vi "Controller Open Ethercat Variables.vi"(8 "error in (no error)":errorcluster, 11 "FOFB Configuration":T3={"FOFB Parameters"={"Network"={"FOFB Controller IP"="", "LNLS Control Network IP"="", "LNLS Control Network Power Supplies TCP Port"=0, "LNLS Control Network FOFB Configuration TCP Port"=0, "LNLS Control Network BPMs TCP Port"=0, "Monitoring Data TCP Port"=0, "Fast Archiver TCP Port"=0, "Fast Command TCP Port"=0, "TCP Listening Timeout"=0}, "Fast Acquisition"={"Sampling Period"=0, "Data Buffer Size"=0, "Monitoring Period"=0}, "Acquisition Network"=[], "Actuation Network"=[]}, "Number of Acquisition Chassis"=0, "Number of Actuation Chassis"=0, "Number of BPM Readings"=0, "BPM Reading Names"=[], "Selected BPM Readings"=[0, 1, 2, 3, 4, 5, 6, 7, 8, 9, 10, 11, 12, 13, 14, 15, 16, 17, 18, 19, 20, 21, 22, 23, 24, 25, 26, 27, 28, 29, 30, 31, 32, 33, 34, 35, 36, 37, 38, 39, 40, 41, 42, 43, 44, 45, 46, 47, 48, 49], "Number of Correctors"=0, "Corrector Names"=[], "Selected Correctors"=[0, 1, 2, 3, 4, 5, 6, 7, 8, 9, 10, 11, 12, 13, 14, 15, 16, 17, 18, 19, 20, 21, 22, 23, 24, 25, 26, 27, 28, 29, 30, 31, 32, 33, 34, 35, 36, 37, 38, 39, 40, 41, 42, 43, 44, 45, 46, 47, 48, 49], "Response Matrix"=[], "Reference Orbit"=[], "Correction Matrix"=[], "FPGA Filter Sets"=[], "Acquisition Chassis Names"=[], "Actuation Chassis Names"=[], "Acquisition Variables"=[], "Actuation Variables"=[], "PS Matrix Mapping"=[], "Inverse PS Matrix Mapping"=[], "BPM Matrix Mapping"=[], "Inverse BPM Matrix Mapping"=[], "BPM Planes"=[], "Corrector Planes"=[]}) -> (0 "error out":errorcluster, 2 "PS Variables":T1, 3 "BPM Variables":T2)   [LabVIEW 2011, in "Controller VIs.lvlib"]
doc: "Open references for all Acquisition and Actuation variables which are used to exchange data between the FOFB Controller and the Acquisition/Actuation chassis via the EtherCAT networks."
uses:
  Controller VIs.lvlib
  Types Definitions/Type FOFB Configuration.ctl
  Types Definitions/Type FOFB Parameters.ctl
  Types Definitions/Type Network Configuration.ctl
  Types Definitions/Type FA Configuration.ctl
  Types Definitions/Type Acquisition Network Configuration.ctl
  Types Definitions/Type Actuation Network Configuration.ctl
  Types Definitions/Type BPM Variables.ctl
  Types Definitions/Type PS Variables.ctl
  Type Definitions.lvlib
  XML VIs.lvlib
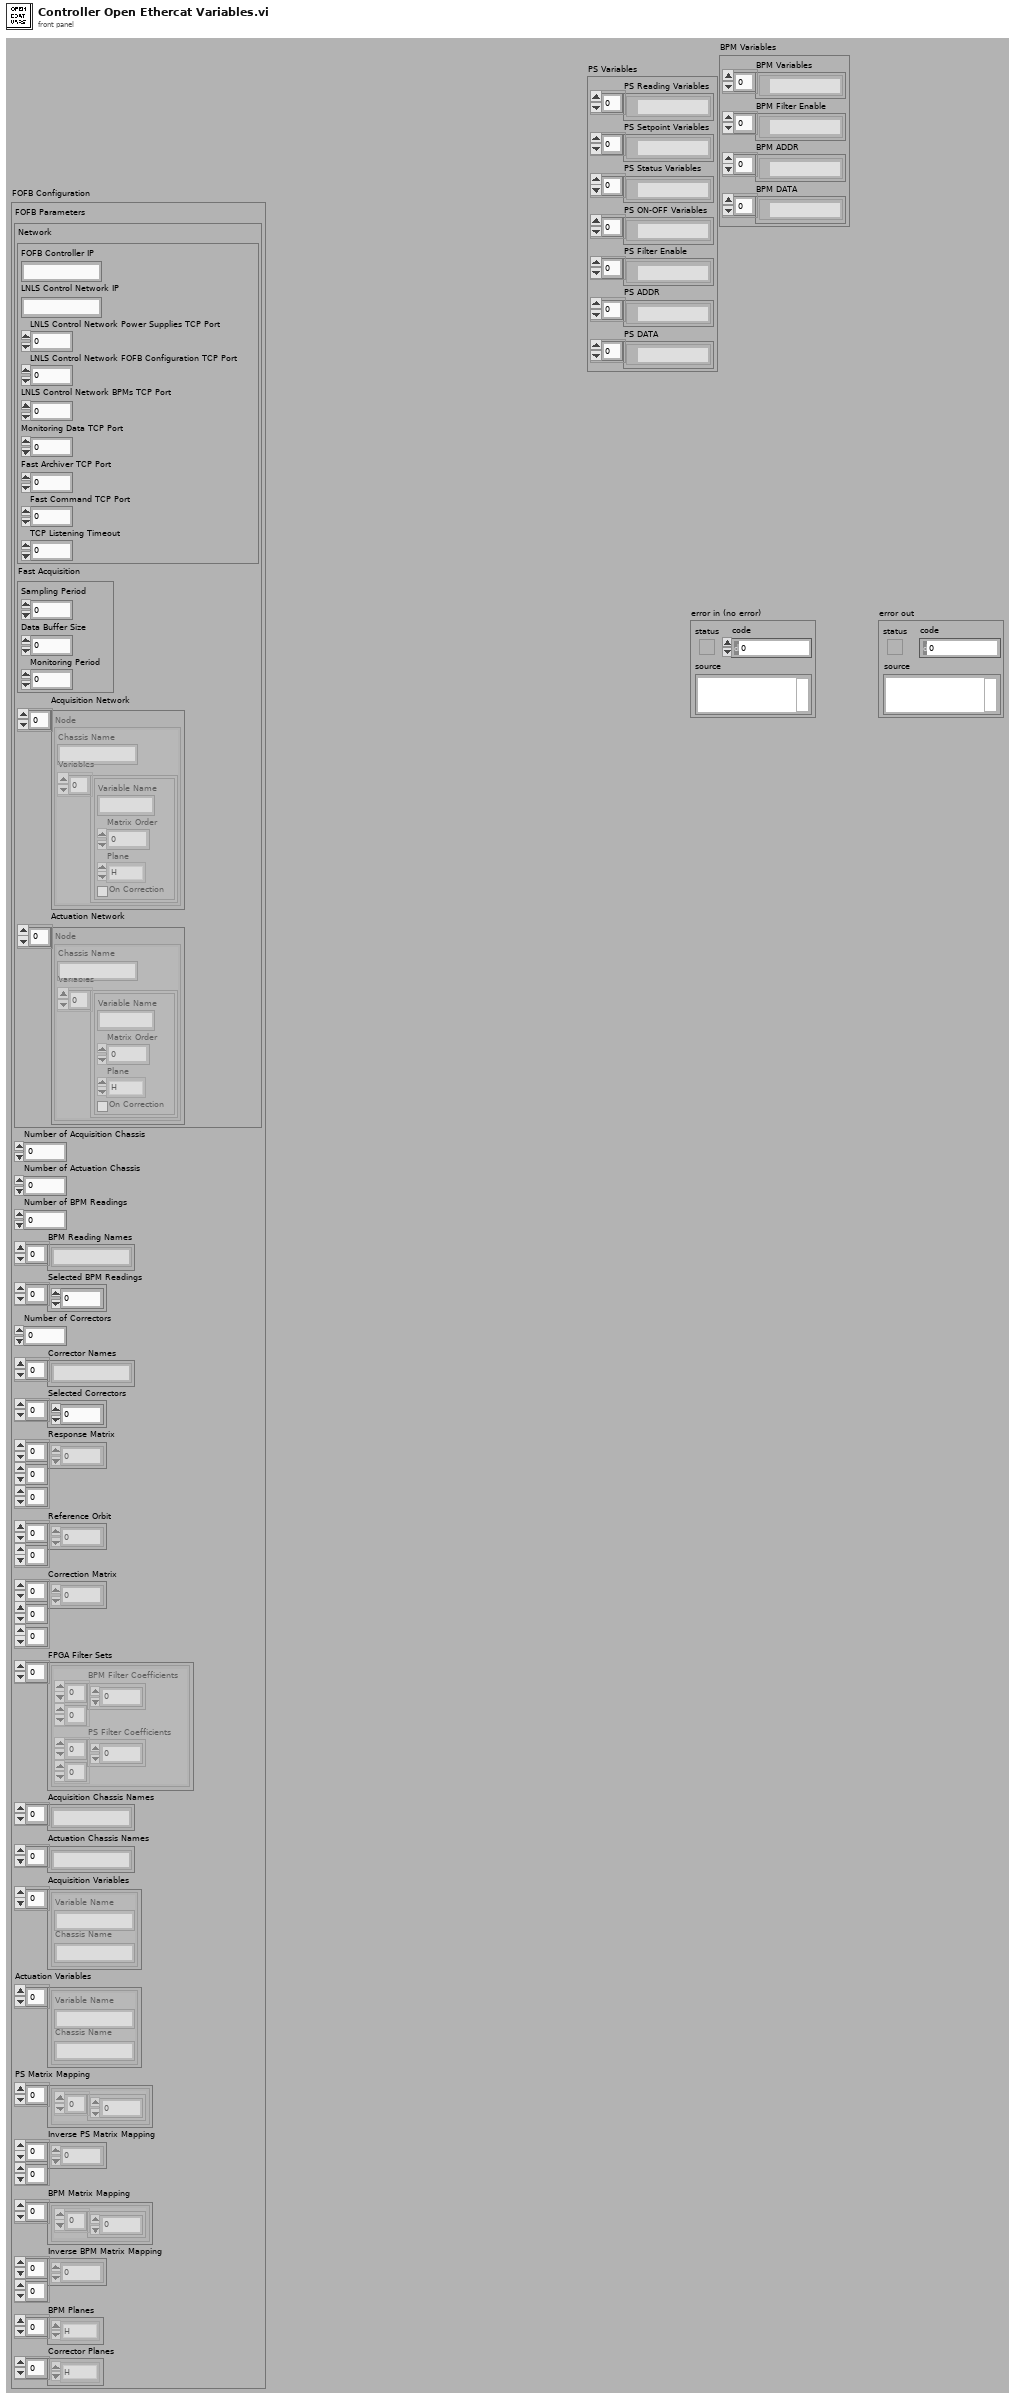
[diagram p1: front panel]
types:
  T1 = typedef "Type Definitions.lvlib/Type PS Variables.ctl" = cluster{"PS Reading Variables":refnum<k21>[], "PS Setpoint Variables":refnum<k21>[], "PS Status Variables":refnum<k21>[], "PS ON-OFF Variables":refnum<k21>[], "PS Filter Enable":refnum<k21>[], "PS ADDR":refnum<k21>[], "PS DATA":refnum<k21>[]}
  T2 = typedef "Type Definitions.lvlib/Type BPM Variables.ctl" = cluster{"BPM Variables":refnum<k21>[], "BPM Filter Enable":refnum<k21>[], "BPM ADDR":refnum<k21>[], "BPM DATA":refnum<k21>[]}
  T3 = typedef "Type Definitions.lvlib/Type FOFB Configuration.ctl" = cluster{"FOFB Parameters":T4, "Number of Acquisition Chassis":i32, "Number of Actuation Chassis":i32, "Number of BPM Readings":i32, "BPM Reading Names":string[], "Selected BPM Readings":u32[], "Number of Correctors":i32, "Corrector Names":string[], "Selected Correctors":u32[], "Response Matrix":dbl[][][], "Reference Orbit":dbl[][], "Correction Matrix":dbl[][][], "FPGA Filter Sets":cluster{"BPM Filter Coefficients":dbl[][], "PS Filter Coefficients":dbl[][]}[], "Acquisition Chassis Names":string[], "Actuation Chassis Names":string[], "Acquisition Variables":cluster{"Variable Name":string, "Chassis Name":string}[], "Actuation Variables":cluster{"Variable Name":string, "Chassis Name":string}[], "PS Matrix Mapping":cluster{u32[]}[], "Inverse PS Matrix Mapping":u32[][], "BPM Matrix Mapping":cluster{u32[]}[], "Inverse BPM Matrix Mapping":u32[][], "BPM Planes":enum8{"H", "V"}[], "Corrector Planes":enum8{"H", "V"}[]}
  T4 = typedef "Type Definitions.lvlib/Type FOFB Parameters.ctl" = cluster{"Network":T5, "Fast Acquisition":T6, "Acquisition Network":T7, "Actuation Network":T8}
  T5 = typedef "Type Definitions.lvlib/Type Network Configuration.ctl" = cluster{"FOFB Controller IP":string, "LNLS Control Network IP":string, "LNLS Control Network Power Supplies TCP Port":u16, "LNLS Control Network FOFB Configuration TCP Port":u16, "LNLS Control Network BPMs TCP Port":u16, "Monitoring Data TCP Port":u16, "Fast Archiver TCP Port":u16, "Fast Command TCP Port":u16, "TCP Listening Timeout":i32}
  T6 = typedef "Type Definitions.lvlib/Type FA Configuration.ctl" = cluster{"Sampling Period":u32, "Data Buffer Size":u32, "Monitoring Period":u32}
  T7 = typedef "Type Definitions.lvlib/Type Acquisition Network Configuration.ctl" = cluster{"Chassis Name":string, "Variables":cluster{"Variable Name":string, "Matrix Order":u32, "Plane":enum8{"H", "V"}, "On Correction":bool}[]}[]
  T8 = typedef "Type Definitions.lvlib/Type Actuation Network Configuration.ctl" = cluster{"Chassis Name":string, "Variables":cluster{"Variable Name":string, "Matrix Order":u32, "Plane":enum8{"H", "V"}, "On Correction":bool}[]}[]
  T9 = cluster{"Variable Name":string, "Chassis Name":string}[]
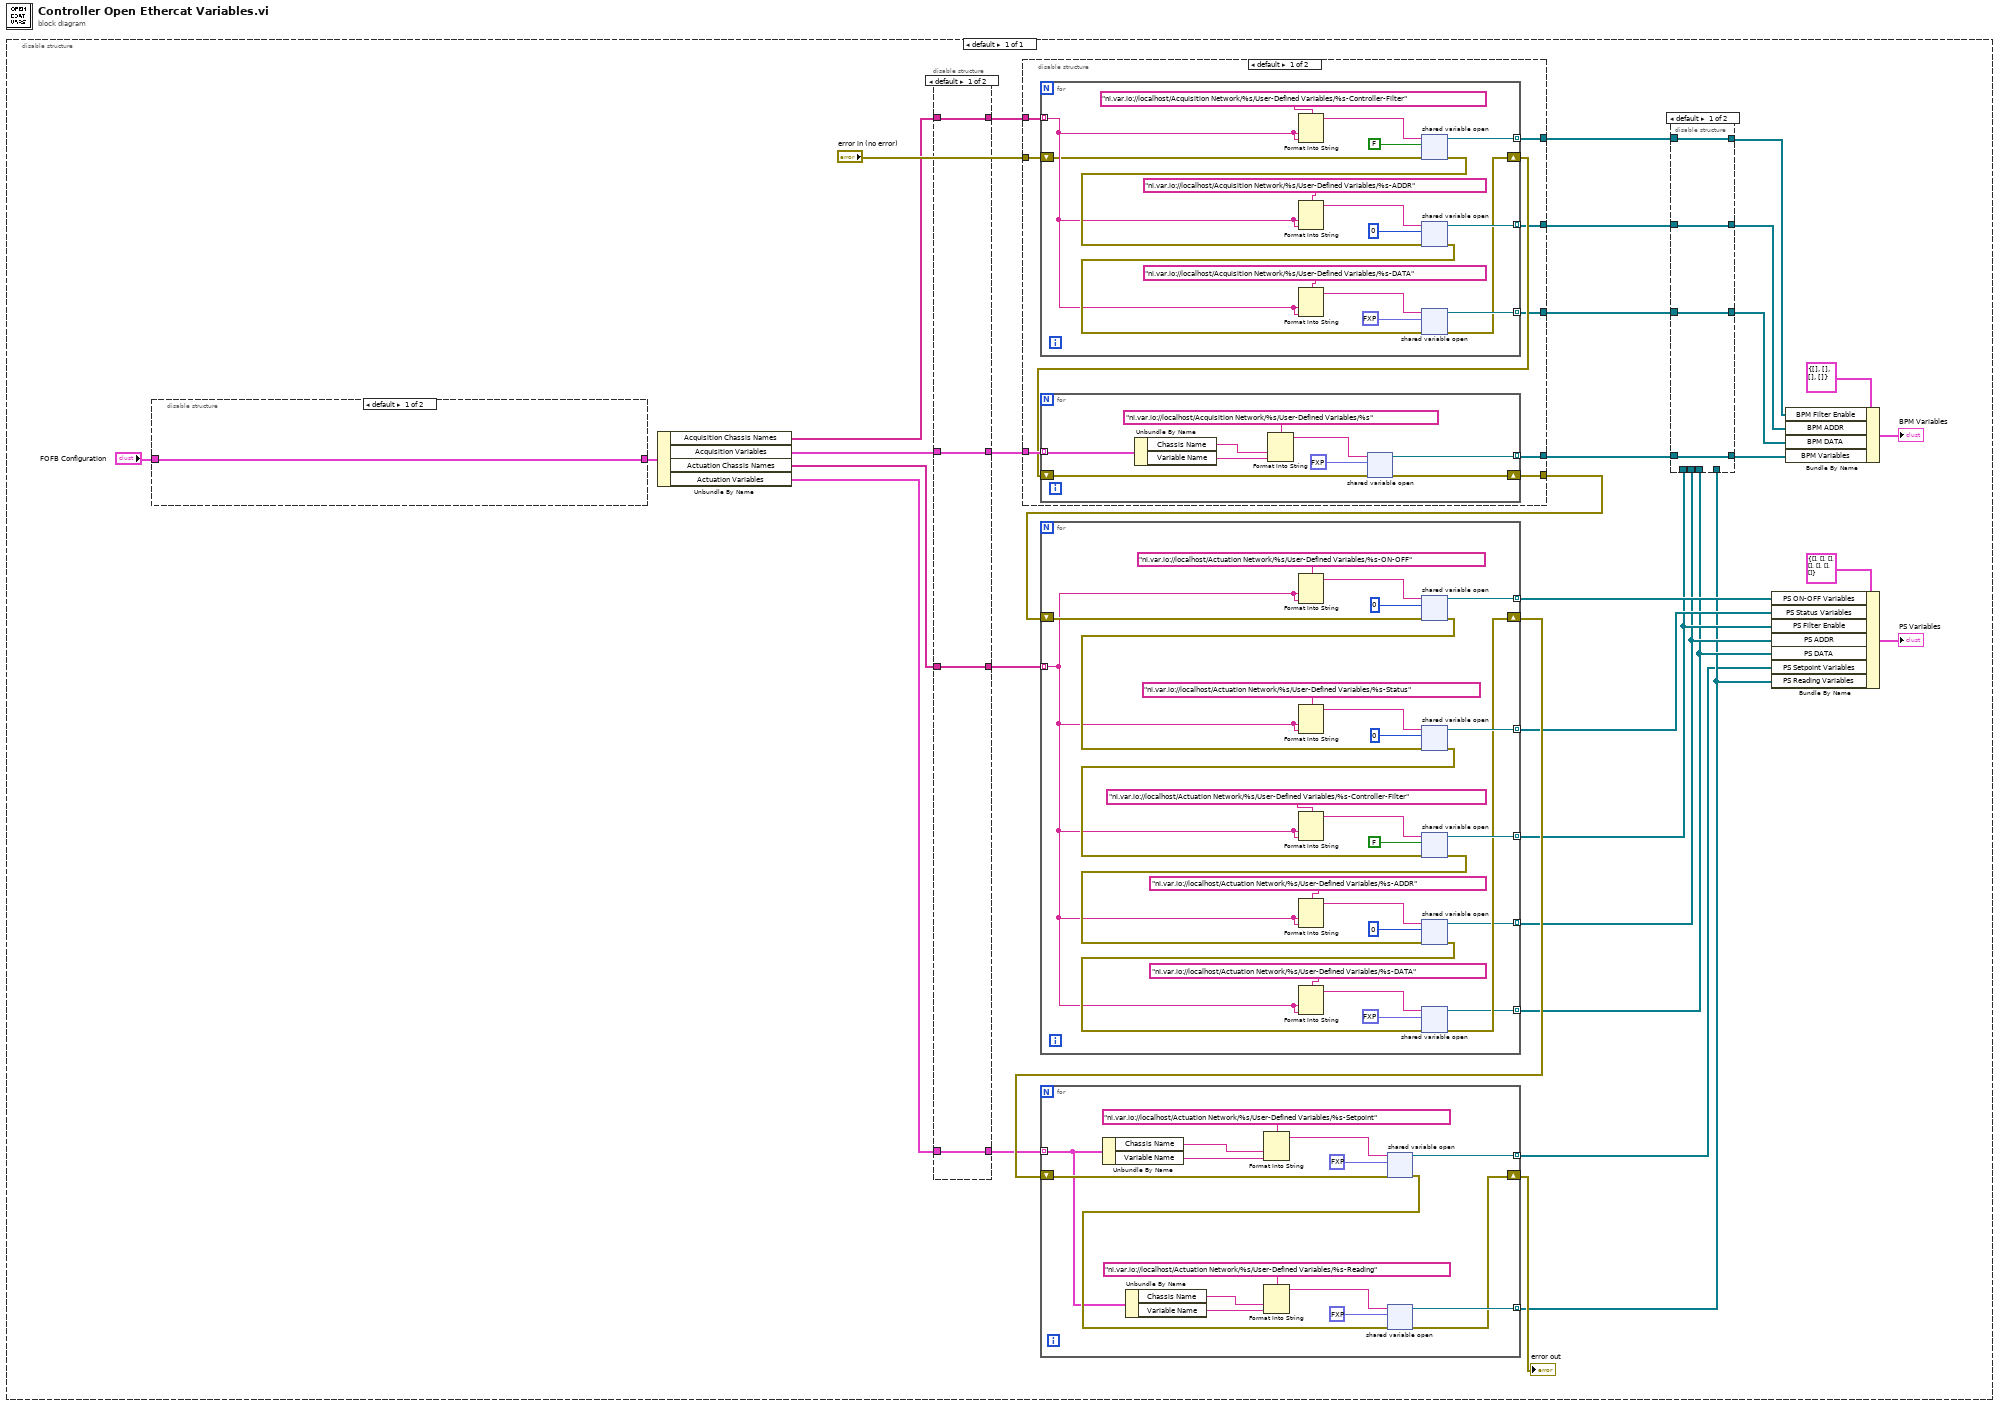
[diagram p0: block diagram]
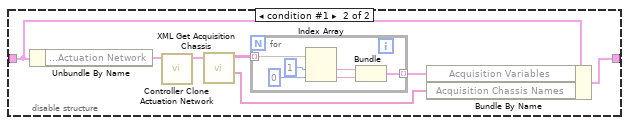
[diagram p2: hidden frame]
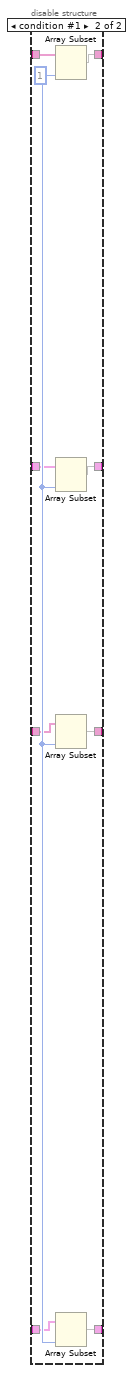
[diagram p3: hidden frame]
diagram:
  n1 = disable-structure shown="default" {
    frame Enabled {
      n2 = disable-structure shown="default" {
        disable-tunnel: "FOFB Configuration" -> [w34 w39]
        disable-tunnel: [w34 w36] -> w1
        frame condition #0 (active) {
        }
        frame condition #1 {
          n3 = Unbundle By Name(w39) -> ("FOFB Parameters.Actuation Network"=w41:T8)
          n4 = call "Controller Clone Actuation Network.vi"("Actuation Network"=w41) -> ("Acquisition Network"=w40:T7)  [unwired: 10 in]
          n5 = call "XML Get Acquisition Chassis.vi"("Acquisition Network"=w40) -> ("Acquisition Chassis Names"=w35:string[], "Acquisition Variable Names"=w38:string[][])  [unwired: 4 in, 5 out]
          n6 = for {
            tunnel: w38 -> [w46] mode=indexing
            tunnel: [w45] -> w37 mode=indexing
            n7 = Index Array(array=w46, index #1=1 ("index"), index #2=0 ("index")) -> (element #1=w42:string, element #2=w44:string)
            n8 = Bundle(w42, w44) -> (w45:cluster{string, string})  [unwired: 1 in]
          }
          n9 = Bundle By Name(cluster=w39, "Acquisition Variables"=w37, "Acquisition Chassis Names"=w35) -> (w36:T3)
        }
      }
      n10 = Unbundle By Name(w1) -> ("Acquisition Chassis Names"=w10:string[], "Acquisition Variables"=w8:T9, "Actuation Chassis Names"=w6:string[], "Actuation Variables"=w4:T9)
      n11 = disable-structure shown="default" {
        disable-tunnel: [w51 w59] -> w9
        disable-tunnel: w10 -> [w51 w60]
        disable-tunnel: [w50 w58] -> w7
        disable-tunnel: w8 -> [w50 w54]
        disable-tunnel: [w48 w57] -> w5
        disable-tunnel: [w49 w56] -> w3
        disable-tunnel: w4 -> [w49 w53]
        disable-tunnel: w6 -> [w48 w52]
        frame condition #0 (active) {
        }
        frame condition #1 {
          w55 = 1 ("length")
          n12 = Array Subset(array=w60, length=w55) -> (w59:string[])  [unwired: 1 in]
          n13 = Array Subset(array=w54, length=w55) -> (w58:T9)  [unwired: 1 in]
          n14 = Array Subset(array=w52, length=w55) -> (w57:string[])  [unwired: 1 in]
          n15 = Array Subset(array=w53, length=w55) -> (w56:T9)  [unwired: 1 in]
        }
      }
      n16 = disable-structure shown="default" {
        disable-tunnel: [w77 w104] -> w30
        disable-tunnel: w7 -> [w76 _]
        disable-tunnel: [w75 _] -> w25
        disable-tunnel: w9 -> [w74 _]
        disable-tunnel: "error in (no error)" -> [w73 w104]
        disable-tunnel: [w71 _] -> w20
        disable-tunnel: [w70 _] -> w19
        disable-tunnel: [w69 _] -> w18
        frame condition #0 (active) {
          n17 = for {
            shift-right: [w78] -> w72
            shift-left: w73 -> [w79]
            tunnel: w74 -> [w84] mode=indexing
            tunnel: [w94] -> w71 mode=indexing
            tunnel: [w81] -> w70 mode=indexing
            tunnel: [w80] -> w69 mode=indexing
            n18 = Format Into String(format string="ni.var.io://localhost/Acquisition Network/%s/User-Defined Variables/%s-Controller-Filter", w84, w84) -> (resulting string=w92:string)  [unwired: 2 in, 1 out]
            n19 = Format Into String(format string="ni.var.io://localhost/Acquisition Network/%s/User-Defined Variables/%s-ADDR", w84, w84) -> (resulting string=w90:string)  [unwired: 2 in, 1 out]
            n20 = Format Into String(format string="ni.var.io://localhost/Acquisition Network/%s/User-Defined Variables/%s-DATA", w84, w84) -> (resulting string=w87:string)  [unwired: 2 in, 1 out]
            n21 = shared-variable-open(w92, w79, FALSE) -> (w94:refnum<k21>, w85:errorcluster)  [unwired: 1 in]
            n22 = shared-variable-open(w90, w85, u16 0) -> (w81:refnum<k21>, w86:errorcluster)  [unwired: 1 in]
            n23 = shared-variable-open(w87, w86, fxp<+/-,22,4> 0.0) -> (w80:refnum<k21>, w78:errorcluster)  [unwired: 1 in]
          }
          n24 = for {
            tunnel: w76 -> [w97] mode=indexing
            shift-right: [w102] -> w77
            shift-left: w72 -> [w101]
            tunnel: [w100] -> w75 mode=indexing
            n25 = Unbundle By Name(w97) -> ("Chassis Name"=w96:string, "Variable Name"=w95:string)
            n26 = Format Into String(format string="ni.var.io://localhost/Acquisition Network/%s/User-Defined Variables/%s", w96, w95) -> (resulting string=w99:string)  [unwired: 2 in, 1 out]
            n27 = shared-variable-open(w99, w101, fxp<+/-,20,5> 0.0 ("BPM Data")) -> (w100:refnum<k21>, w102:errorcluster)  [unwired: 1 in]
          }
        }
        frame condition #1 {
        }
      }
      n28 = for {
        shift-right: [w112] -> w29
        shift-left: w30 -> [w124]
        tunnel: w5 -> [w109] mode=indexing
        tunnel: [w123] -> w17 mode=indexing
        tunnel: [w122] -> w16 mode=indexing
        tunnel: [w120] -> w15 mode=indexing
        tunnel: [w106] -> w14 mode=indexing
        tunnel: [w105] -> w13 mode=indexing
        n29 = Format Into String(format string="ni.var.io://localhost/Actuation Network/%s/User-Defined Variables/%s-ON-OFF", w109, w109) -> (resulting string=w131:string)  [unwired: 2 in, 1 out]
        n30 = Format Into String(format string="ni.var.io://localhost/Actuation Network/%s/User-Defined Variables/%s-Status", w109, w109) -> (resulting string=w128:string)  [unwired: 2 in, 1 out]
        n31 = Format Into String(format string="ni.var.io://localhost/Actuation Network/%s/User-Defined Variables/%s-Controller-Filter", w109, w109) -> (resulting string=w118:string)  [unwired: 2 in, 1 out]
        n32 = Format Into String(format string="ni.var.io://localhost/Actuation Network/%s/User-Defined Variables/%s-ADDR", w109, w109) -> (resulting string=w116:string)  [unwired: 2 in, 1 out]
        n33 = Format Into String(format string="ni.var.io://localhost/Actuation Network/%s/User-Defined Variables/%s-DATA", w109, w109) -> (resulting string=w113:string)  [unwired: 2 in, 1 out]
        n34 = shared-variable-open(w131, w124, u8 0) -> (w123:refnum<k21>, w127:errorcluster)  [unwired: 1 in]
        n35 = shared-variable-open(w128, w127, u8 0) -> (w122:refnum<k21>, w121:errorcluster)  [unwired: 1 in]
        n36 = shared-variable-open(w118, w121, FALSE) -> (w120:refnum<k21>, w110:errorcluster)  [unwired: 1 in]
        n37 = shared-variable-open(w116, w110, u16 0) -> (w106:refnum<k21>, w111:errorcluster)  [unwired: 1 in]
        n38 = shared-variable-open(w113, w111, fxp<+/-,22,4> 0.0) -> (w105:refnum<k21>, w112:errorcluster)  [unwired: 1 in]
      }
      n39 = for {
        shift-right: [w137] -> w31
        shift-left: w29 -> [w138]
        tunnel: w3 -> [w134] mode=indexing
        tunnel: [w142] -> w11 mode=indexing
        tunnel: [w141] -> w12 mode=indexing
        n40 = Unbundle By Name(w134) -> ("Chassis Name"=w136:string, "Variable Name"=w135:string)
        n41 = Unbundle By Name(w134) -> ("Chassis Name"=w132:string, "Variable Name"=w133:string)
        n42 = Format Into String(format string="ni.var.io://localhost/Actuation Network/%s/User-Defined Variables/%s-Setpoint", w136, w135) -> (resulting string=w147:string)  [unwired: 2 in, 1 out]
        n43 = Format Into String(format string="ni.var.io://localhost/Actuation Network/%s/User-Defined Variables/%s-Reading", w132, w133) -> (resulting string=w144:string)  [unwired: 2 in, 1 out]
        n44 = shared-variable-open(w147, w138, fxp<+/-,20,5> 0.0 ("PS Setpoint Data")) -> (w142:refnum<k21>, w143:errorcluster)  [unwired: 1 in]
        n45 = shared-variable-open(w144, w143, fxp<+/-,20,5> 0.0 ("PS Reading Data")) -> (w141:refnum<k21>, w137:errorcluster)  [unwired: 1 in]
      }
      "error out" <- w31
      n46 = disable-structure shown="default" {
        disable-tunnel: [w64 w68] -> w26
        disable-tunnel: w12 -> [_ w68]
        disable-tunnel: w25 -> [w64 _]
        disable-tunnel: w13 -> [_ w67]
        disable-tunnel: w14 -> [_ w66]
        disable-tunnel: w15 -> [_ w65]
        disable-tunnel: [w61 w67] -> w23
        disable-tunnel: [w62 w66] -> w22
        disable-tunnel: [w63 w65] -> w21
        disable-tunnel: w20 -> [w63 _]
        disable-tunnel: w19 -> [w62 _]
        disable-tunnel: w18 -> [w61 _]
        frame condition #0 (active) {
        }
        frame condition #1 {
        }
      }
      n47 = Bundle By Name(cluster=T1 {"PS Reading Variables"=[], "PS Setpoint Variables"=[], "PS Status Variables"=[], "PS ON-OFF Variables"=[], "PS Filter Enable"=[], "PS ADDR"=[], "PS DATA"=[]} ("output cluster"), "PS ON-OFF Variables"=w17, "PS Status Variables"=w16, "PS Filter Enable"=w15, "PS ADDR"=w14, "PS DATA"=w13, "PS Setpoint Variables"=w11, "PS Reading Variables"=w12) -> (→"PS Variables":T1)
      n48 = Bundle By Name(cluster=T2 {"BPM Variables"=[], "BPM Filter Enable"=[], "BPM ADDR"=[], "BPM DATA"=[]} ("output cluster"), "BPM Filter Enable"=w21, "BPM ADDR"=w22, "BPM DATA"=w23, "BPM Variables"=w26) -> (→"BPM Variables":T2)
    }
  }
